vi "After Launch Init Core.vi"(8 "error in (no error)":errorcluster, 11 "KIT-QVA in":refnum<class "KIT-QVA.lvclass">) -> (0 "error out":errorcluster, 3 "KIT-QVA out":refnum<class "KIT-QVA.lvclass">)   [LabVIEW 2014, in "KIT-QVA.lvlib" / "KIT-QVA.lvclass"]
doc: "Use <b>Pre Launch init.vi</b> method for sanity checks that are supposed to prevent the actor from launching if they fail. Use <B>this</B> method instead to initialize this actor when it has been activated. A corresponding high priority message will become dispatched before the <B>Actor Core.vi</b> is called.\n\n<b>Derived classed should call the parent methode first</b> and their own initialization code after.\n\nRefer also to the ongoing discussion at https://decibel.ni.com/content/message/57394#57394."
uses:
  KIT-QVA.lvclass
  CSPP_Core/Classes/CS++ProcessVariables/ProcessVariable/PV.lvclass
  KIT-QVA.lvclass/KIT-QVA.ctl
  CSPP_Core/Classes/CS++ProcessVariables/ProcessVariable/PV.lvclass/PV.ctl
  <vilib>/ActorFramework/Actor/Actor.lvclass/Actor.ctl
  <vilib>/ActorFramework/Message Enqueuer/Message Enqueuer.lvclass/Message Enqueuer.ctl
  CSPP_Core/Classes/CS++ProcessVariables/ProcessVariable/Write Data.vi
  CSPP_Core/Classes/CS++ProcessVariables/ProcessVariable/Write Error.vi
  CSPP_Core/Classes/CS++ProcessVariables/ProcessVariable/Write Quality.vi
  CSPP_Core/Classes/CS++ProcessVariables/ProcessVariable/Write status.vi
  CSPP_Core/Classes/CS++ProcessVariables/ProcessVariable/Write Timestamp.vi
  <vilib>/ActorFramework/Message Enqueuer/Init from Existing Queue.vi
  <vilib>/ActorFramework/Message Enqueuer/Enqueue.vi
  <vilib>/ActorFramework/Message Priority Queue/Priority Enqueue.vi
  <vilib>/ActorFramework/Message Enqueuer/Message Enqueuer.lvclass
  KIT-QVA Messages/Read Status Msg/Read Status Msg.lvclass
  CSPP_Core/Actors/CS++DeviceActor/CS++DeviceActor.lvclass
  CSPP_Core/Classes/CS++ProcessVariables/PVConnection/PVConnection.lvclass
  <vilib>/ActorFramework/Actor/Actor.lvclass
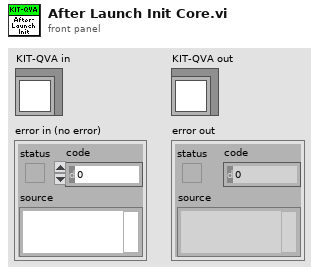
[diagram p1: front panel]
types:
  T1 = cluster{"Read Access":enum8{"Allowed", "Required", "None"}, "Write Access":enum8{"Allowed", "Required", "None"}}
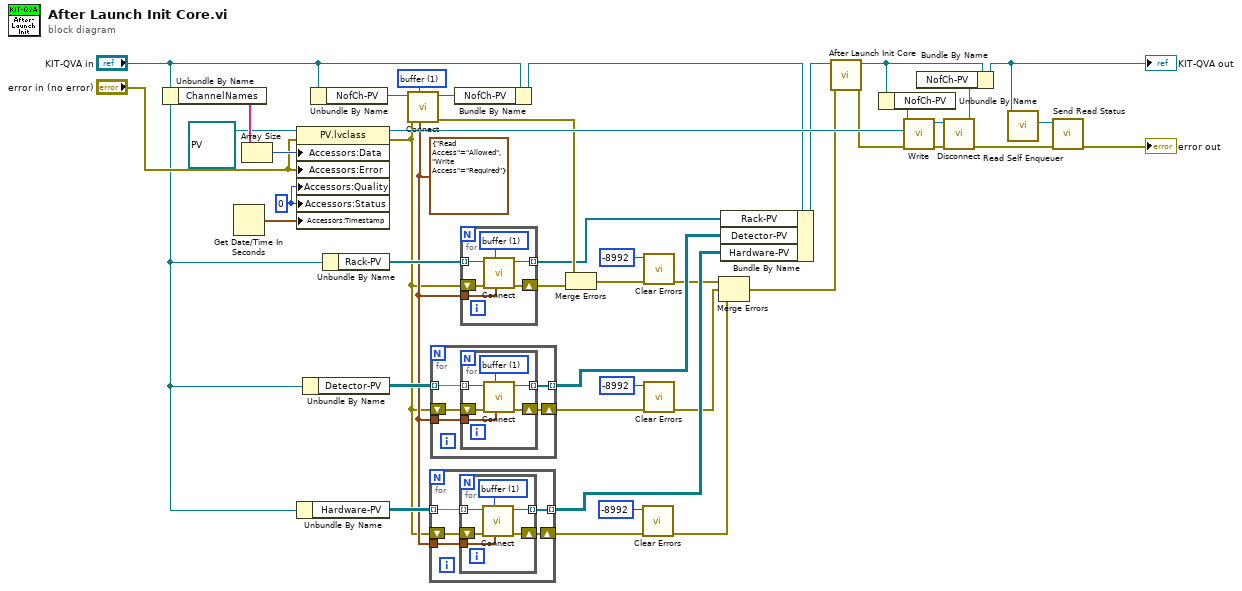
[diagram p0: block diagram]
diagram:
  w33 = u16 1 items=["commit", "buffer"] ("Mode (commit)")
  w8 = T1 {"Read Access"=enum."Allowed", "Write Access"=enum."Required"} ("Access (R/W allowed)")
  w40 = 0 ("Quality")
  n1 = Unbundle By Name("KIT-QVA in") -> ("ChannelNames"=w43:string[])
  n2 = Get Date/Time In Seconds() -> (seconds since 1Jan1904=w39:timestamp)
  n3 = Array Size(array=w43) -> (size(s)=w41:i32)
  n4 = property class="PV.lvclass"(reference=refnum<class "PV.lvclass"> refnum ("CS++ProcessVariables.lvlib:PV.lvclass"), error in="error in (no error)", "Accessors:Data"=w41, "Accessors:Error"="error in (no error)", "Accessors:Quality"=w40, "Accessors:Status"=w40, "Accessors:Timestamp"=w39) -> (reference out=w35:refnum<class "PV.lvclass">, error out=w7:errorcluster)
  n5 = Unbundle By Name("KIT-QVA in") -> ("Hardware-PV"=w17:refnum<class "PVConnection.lvclass">[][])
  n6 = Unbundle By Name("KIT-QVA in") -> ("Detector-PV"=w20:refnum<class "PVConnection.lvclass">[][])
  n7 = Unbundle By Name("KIT-QVA in") -> ("NofCh-PV"=w38:refnum<class "PVConnection.lvclass">)
  n8 = Unbundle By Name("KIT-QVA in") -> ("Rack-PV"=w24:refnum<class "PVConnection.lvclass">[])
  n9 = call "Connect.vi"("Access (R/W allowed)"=w8, "Mode (buffer)"=w33, "Error In"=w7, "PVConnection in"=w38) -> ("Error Out"=w31:errorcluster, "PVConnection out"=w28:refnum<class "PVConnection.lvclass">)  [unwired: 6 in]
  n10 = for {
    tunnel: w8 -> [w48]
    tunnel: w17 -> [w47] mode=indexing
    tunnel: [w46] -> w15 mode=indexing
    shift-right: [w45] -> w5
    shift-left: w7 -> [w44]
    n11 = for {
      tunnel: w47 -> [w54] mode=indexing
      tunnel: [w53] -> w46 mode=indexing
      tunnel: w48 -> [w52]
      shift-right: [w51] -> w45
      shift-left: w44 -> [w50]
      w49 = u16 1 items=["commit", "buffer"] ("Mode (commit)")
      n12 = call "Connect.vi"("Access (R/W allowed)"=w52, "Mode (buffer)"=w49, "Error In"=w50, "PVConnection in"=w54) -> ("Error Out"=w51:errorcluster, "PVConnection out"=w53:refnum<class "PVConnection.lvclass">)  [unwired: 6 in]
    }
  }
  n13 = for {
    tunnel: w8 -> [w59]
    tunnel: w20 -> [w58] mode=indexing
    tunnel: [w57] -> w16 mode=indexing
    shift-right: [w56] -> w6
    shift-left: w7 -> [w55]
    n14 = for {
      tunnel: w58 -> [w65] mode=indexing
      tunnel: [w64] -> w57 mode=indexing
      tunnel: w59 -> [w63]
      shift-right: [w62] -> w56
      shift-left: w55 -> [w61]
      w60 = u16 1 items=["commit", "buffer"] ("Mode (commit)")
      n15 = call "Connect.vi"("Access (R/W allowed)"=w63, "Mode (buffer)"=w60, "Error In"=w61, "PVConnection in"=w65) -> ("Error Out"=w62:errorcluster, "PVConnection out"=w64:refnum<class "PVConnection.lvclass">)  [unwired: 6 in]
    }
  }
  n16 = Bundle By Name(cluster="KIT-QVA in", "NofCh-PV"=w28) -> (w23:refnum<class "KIT-QVA.lvclass">)
  n17 = for {
    tunnel: w24 -> [w71] mode=indexing
    tunnel: [w70] -> w21 mode=indexing
    tunnel: w8 -> [w69]
    shift-right: [w68] -> w30
    shift-left: w7 -> [w67]
    w66 = u16 1 items=["commit", "buffer"] ("Mode (commit)")
    n18 = call "Connect.vi"("Access (R/W allowed)"=w69, "Mode (buffer)"=w66, "Error In"=w67, "PVConnection in"=w71) -> ("Error Out"=w68:errorcluster, "PVConnection out"=w70:refnum<class "PVConnection.lvclass">)  [unwired: 6 in]
  }
  n19 = Merge Errors(w31, w30) -> (w29:errorcluster)
  n20 = call <vilib>:"Clear Errors.vi"("error in (no error)"=w5, "specific error code to clear (0: all)"=-8992) -> ("error out"=w13:errorcluster)  [unwired: 4 in, 1 out]
  n21 = call <vilib>:"Clear Errors.vi"("error in (no error)"=w29, "specific error code to clear (0: all)"=-8992) -> ("error out"=w12:errorcluster)  [unwired: 4 in, 1 out]
  n22 = call <vilib>:"Clear Errors.vi"("error in (no error)"=w6, "specific error code to clear (0: all)"=-8992) -> ("error out"=w14:errorcluster)  [unwired: 4 in, 1 out]
  n23 = Merge Errors(w12, w14, w13) -> (w11:errorcluster)
  n24 = Bundle By Name(cluster=w23, "Rack-PV"=w21, "Detector-PV"=w16, "Hardware-PV"=w15) -> (w22:refnum<class "KIT-QVA.lvclass">)
  n25 = call-parent "After Launch Init Core.vi"("error in (no error)"=w11, "CS++DeviceActor in"=w22) -> ("error out"=w25:errorcluster, "CS++DeviceActor out"=w32:refnum<class "KIT-QVA.lvclass">)  [unwired: 8 in]
  n26 = Unbundle By Name(w32) -> ("NofCh-PV"=w27:refnum<class "PVConnection.lvclass">)
  n27 = call "Write.vi"("error in (no error)"=w25, "PV"=w35, "PVConnection in"=w27) -> ("error out"=w36:errorcluster, "PVConnection out"=w37:refnum<class "PVConnection.lvclass">)  [unwired: 7 in]
  n28 = call "Disconnect.vi"("error in (no error)"=w36, "PVConnection in"=w37) -> ("error out"=w2:errorcluster, "PVConnection out"=w26:refnum<class "PVConnection.lvclass">)  [unwired: 8 in]
  n29 = Bundle By Name(cluster=w32, "NofCh-PV"=w26) -> (w4:refnum<class "KIT-QVA.lvclass">)
  "KIT-QVA out" <- w4
  n30 = call <vilib>:"Read Self Enqueuer.vi"("Actor"=w4) -> ("Self Enqueuer"=w3:refnum<class "Message Enqueuer.lvclass">)  [unwired: 10 in]
  n31 = call "Send Read Status.vi"("error in (no error)"=w2, "Message Enqueuer"=w3) -> ("error out"=→"error out":errorcluster)  [unwired: 8 in, 1 out]
